vi "Global 1.vi"() -> ()   [LabVIEW 2022 SP3]
panel:
  in  "Boolean":bool
  in  "Pixel count":u32
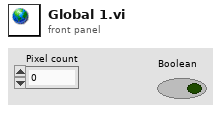
[diagram p1: front panel]
diagram:
